vi "2 - Get start end.vi"() -> ()   [LabVIEW 2013]
uses:
  <vilib>/vision/NI_Vision_Development_Module.lvlib
panel:
  in  "back":bool
  in  "forward":bool
  in  "fast forward":bool
  out "start":i32[](array[numeric])
  out "end":i32[](array[numeric])
  out "end":i32[](array[numeric])
  out "start":i32[](array[numeric])
  in  "start":bool
  in  "End":bool
  out "Number of Frames":u32
  in  "frame jump":i32=3
  in  "speed":u32(slide)
  in  "start":i32(slide) step=219843704 scale=0.0..69408.0
  out "Image 3":T1(plugin-control)
  in  "AVI Path":path=path "E:/PhD work/PhD research work/Videos/Chen Jin vs Hu Yun (Edited).avi"
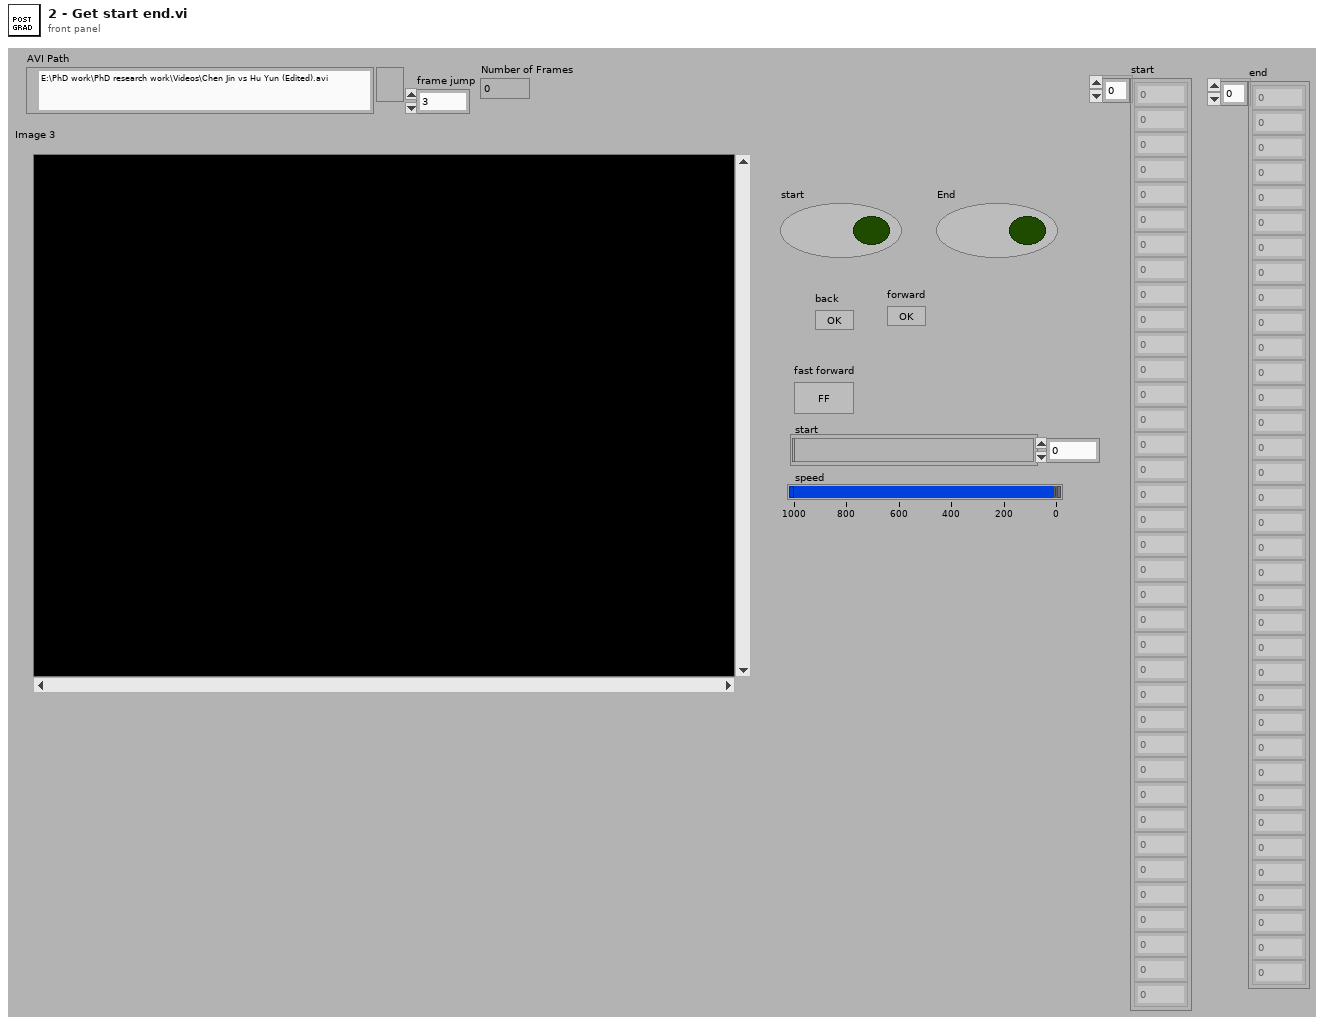
[diagram p1: front panel]
types:
  T1 = typedef "IMAQ Image.ctl" = refnum<image>
  T2 = typedef "Image Type" = u32
  T3 = typedef "AviRefnum.ctl" = refnum<k1>
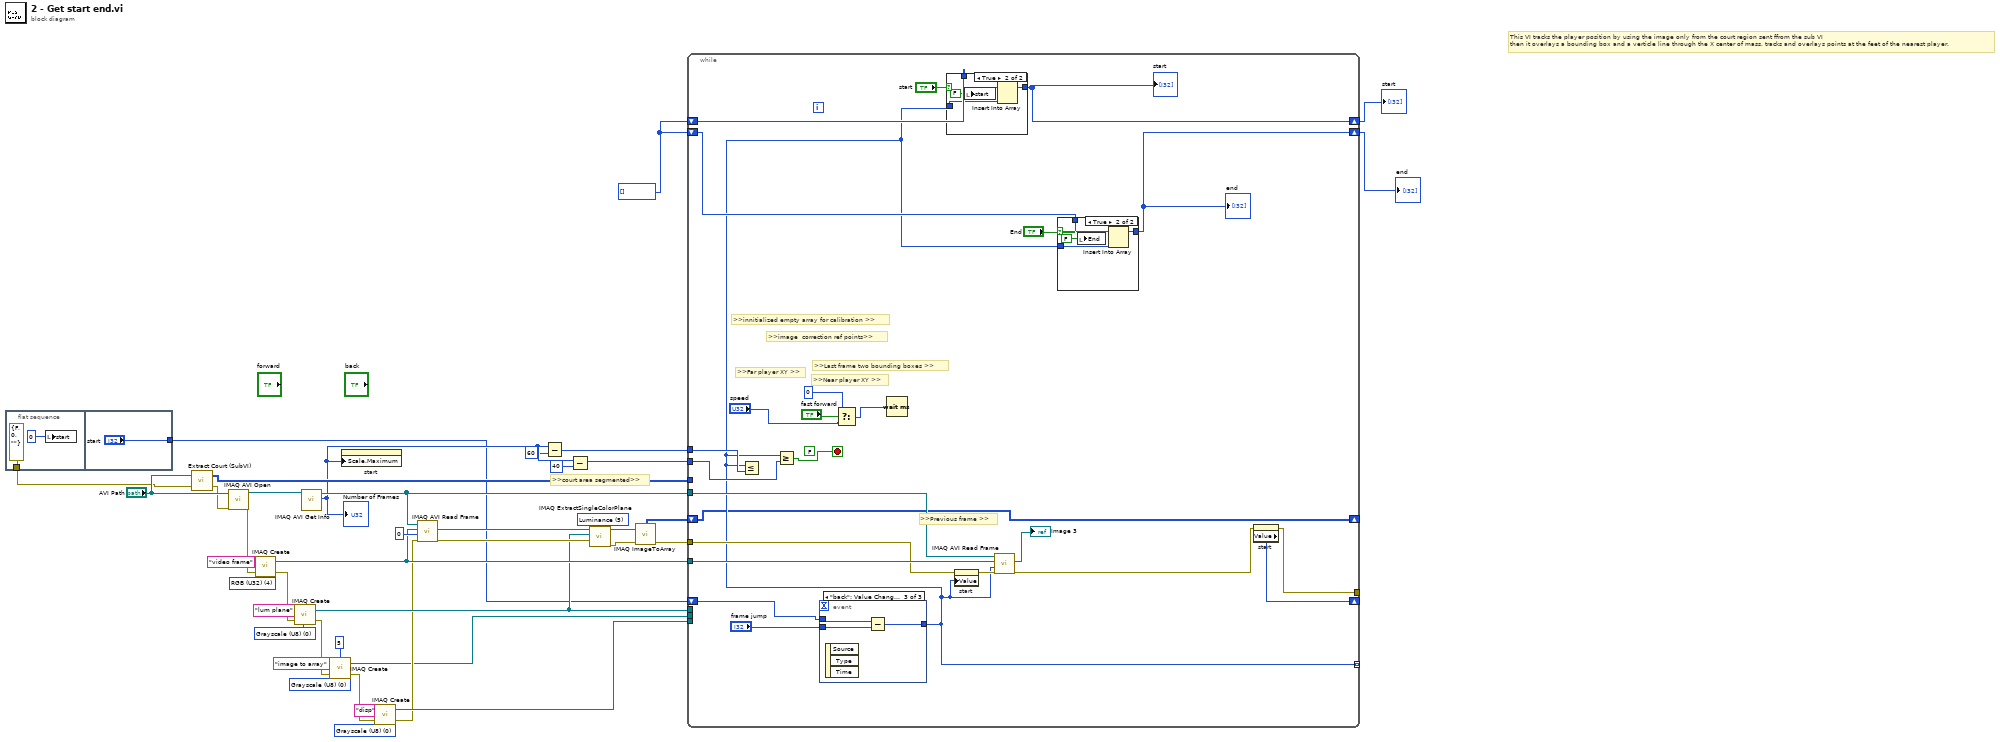
[diagram p0: block diagram]
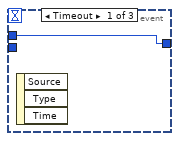
[diagram p2: hidden frame]
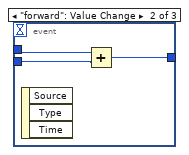
[diagram p3: hidden frame]
diagram:
  w5 = i32[] [] ("input array")
  w26 = T2 0 items=["Grayscale (U8)", "Grayscale (I16)", "Grayscale (SGL)", "Complex (CSG)", "RGB (U32)", "HSL (U32)", "RGB (U64)", "Grayscale (U16)"] ("Image Type")
  w33 = 5 items=["Red", "Green", "Blue", "Hue", "Saturation", "Luminance", "Value", "Intensity"] ("Color Plane")
  w34 = T2 0 items=["Grayscale (U8)", "Grayscale (I16)", "Grayscale (SGL)", "Complex (CSG)", "RGB (U32)", "HSL (U32)", "RGB (U64)", "Grayscale (U16)"] ("Image Type")
  w38 = T2 0 items=["Grayscale (U8)", "Grayscale (I16)", "Grayscale (SGL)", "Complex (CSG)", "RGB (U32)", "HSL (U32)", "RGB (U64)", "Grayscale (U16)"] ("Image Type")
  w36 = T2 4 items=["Grayscale (U8)", "Grayscale (I16)", "Grayscale (SGL)", "Complex (CSG)", "RGB (U32)", "HSL (U32)", "RGB (U64)", "Grayscale (U16)"] ("Image Type")
  # ">>court area segmented>>"
  # "This VI tracks the player position by using the image only from the court region sent ffrom the sub VI\nthen it overlays a bounding box and a verticle line through the X center of mass. tracks and overlays points at the feet of the nearest player."
  n1 = flat-sequence {
    tunnel: [errorcluster {"status"=FALSE, "code"=0, "source"=""} ("error in (no error)")] -> w2
    tunnel: ["start"] -> w1
    frame #0 {
      n2 = local write "start"(0 ("start")) -> ()
    }
    frame #1 {
    }
  }
  n3 = call "Extract Court (SubVI).vi"("error in (no error)"=w2, "AVI Path"="AVI Path") -> ("error out"=w40:errorcluster, "Court pixels out"=w16:u8[][])
  n4 = call "IMAQ AVI Open"("error in (no error)"=w40, "AVI Path"="AVI Path") -> ("error out"=w22:errorcluster, "Avi Refnum"=w14:T3)  [unwired: 8 in]
  n5 = call "IMAQ Create"("Image Name"="video frame", "Image Type"=w36, "error in (no error)"=w22) -> ("New Image"=w30:T1, "error out"=w21:errorcluster)  [unwired: 2 in]
  n6 = call "IMAQ Create"("Image Name"="lum plane", "Image Type"=w38, "error in (no error)"=w21) -> ("New Image"=w29:T1, "error out"=w20:errorcluster)  [unwired: 2 in]
  n7 = call "IMAQ AVI Get Info"("Avi Refnum"=w14) -> ("Number of Frames"=w10:u32, "Avi Refnum (duplicate)"=w13:T3)  [unwired: 6 in, 3 out]
  "Number of Frames" <- w10
  n8 = call "IMAQ Create"("Border Size"=5, "Image Name"="image to array", "Image Type"=w34, "error in (no error)"=w20) -> ("New Image"=w15:T1, "error out"=w19:errorcluster)  [unwired: 1 in]
  n9 = property on="start" class="Slide (strict)"("Scale.Maximum"=w10) -> ()  [unwired: 2 in, 2 out]
  n10 = call "IMAQ Create"("Image Name"="disp", "Image Type"=w26, "error in (no error)"=w19) -> ("New Image"=w24:T1, "error out"=w18:errorcluster)  [unwired: 2 in]
  n11 = call "IMAQ AVI Read Frame"("error in (no error)"=w18, "Frame Number"=u32 0, "Image"=w30, "Avi Refnum"=w13) -> ("error out"=w32:errorcluster, "Image Out"=w11:T1)  [unwired: 4 in, 2 out]
  n12 = Subtract(x=w10, y=u32 60) -> (x-y=w7:u32)
  n13 = Subtract(x=w10, y=u32 40) -> (x-y=w6:u32)
  n14 = call "IMAQ ExtractSingleColorPlane"("Color Plane"=w33, "error in (no error)"=w32, "Image Dst"=w29, "Image Src"=w11) -> ("error out"=w23:errorcluster, "Image Dst Out"=w27:T1)  [unwired: 6 in]
  n15 = call "IMAQ ImageToArray"("error in (no error)"=w23, "Image"=w27) -> ("error out"=w12:errorcluster, "Image Pixels (U8)"=w28:u8[][])  [unwired: 2 in, 3 out]
  n16 = while {
    tunnel: w13 -> [w68]
    tunnel: w30 -> [w69]
    tunnel: w16 -> [_]
    tunnel: w29 -> [_]
    tunnel: w15 -> [_]
    shift-right: [w45] -> _
    shift-left: w28 -> [w45]
    tunnel: w24 -> [_]
    shift-right: [w50] -> _
    shift-left: w1 -> [w48]
    tunnel: w12 -> [w67]
    tunnel: [w65] -> _
    tunnel: w7 -> [w63]
    tunnel: w6 -> [w62]
    tunnel: [w46] -> _ mode=indexing
    shift-right: [w56] -> w3
    shift-left: w5 -> [w57]
    shift-right: [w58] -> w4
    shift-left: w5 -> [w59]
    stop <- w64 stop-if-true
    (unwired) FALSE
    # ">>innitialized empty array for calibration >>"
    # ">>image  correction ref points>>"
    # ">>Last frame two bounding boxes >>"
    # ">>Far player XY >>"
    # ">>Near player XY >>"
    # ">>Previous frame >>"
    n17 = event shown="[2] \"back\": Value Change" {
      selector: _ -> [_ _ _]
      dyn-events: _ -> [_ _ _]
      timeout: _ -> [_ _ _]
      tunnel: w48 -> [w70 w73 w76]
      tunnel: "frame jump" -> [_ w72 w75]
      tunnel: [w70 w71 w74] -> w46
      event Timeout {
        n18 = event-data() -> ()  [unwired: 1 in, 3 out]
      }
      event "forward": Value Change {
        n19 = event-data() -> ()  [unwired: 1 in, 3 out]
        n20 = Add(x=w73, y=w72) -> (x+y=w71:i32)
      }
      event "back": Value Change {
        n21 = event-data() -> ()  [unwired: 1 in, 3 out]
        n22 = Subtract(x=w76, y=w75) -> (x-y=w74:i32)
      }
    }
    n23 = Less Or Equal?(x=w46, y=w63) -> ()  [unwired: 1 out]
    n24 = Greater Or Equal?(x=w46, y=w62) -> (x >= y?=w64:bool)
    n25 = Select(t=u32 0, s="fast forward", f="speed") -> (s? t:f=w52:u32)
    n26 = Wait (ms)(milliseconds to wait=w52) -> ()  [unwired: 1 out]
    n27 = case shown="True" "start" {
      tunnel: w59 -> [w82 w86]
      tunnel: w46 -> [_ w85]
      tunnel: [w82 w84] -> w58
      frame False {
      }
      frame True {
        n28 = local write "start"(FALSE ("start")) -> ()
        n29 = Insert Into Array(array=w86, new element=w85) -> (w84:i32[])  [unwired: 1 in]
      }
    }
    "start" <- w58
    n30 = property on="start" class="Slide (strict)"(error in=w67, "Value"=w46) -> (error out=w66:errorcluster)  [unwired: 1 in, 1 out]
    n31 = call "IMAQ AVI Read Frame"("error in (no error)"=w66, "Frame Number"=w46, "Image"=w69, "Avi Refnum"=w68) -> ("error out"=w49:errorcluster, "Image Out"=→"Image 3":T1)  [unwired: 4 in, 2 out]
    n32 = case shown="True" "End" {
      tunnel: w57 -> [w77 w81]
      tunnel: w46 -> [_ w80]
      tunnel: [w77 w79] -> w56
      frame False {
      }
      frame True {
        n33 = local write "End"(FALSE ("End")) -> ()
        n34 = Insert Into Array(array=w81, new element=w80) -> (w79:i32[])  [unwired: 1 in]
      }
    }
    "end" <- w56
    n35 = property on="start" class="Slide (strict)"(error in=w49) -> (error out=w65:errorcluster, "Value"=w50:i32)  [unwired: 1 in, 1 out]
  }
  "end" <- w3
  "start" <- w4
